vi "Windows.vi"(8 "error in (no error)":errorcluster, 10 "Font in":string, 11 "Font":refnum<vi>) -> (0 "error out":errorcluster, 2 "Font out":string)   [LabVIEW 2020]
uses:
  vi.lib/LabVIEW Icon API/lv_icon/lv_icon.lvlib
  <vilib>/registry/registry.llb/Registry SAM.ctl
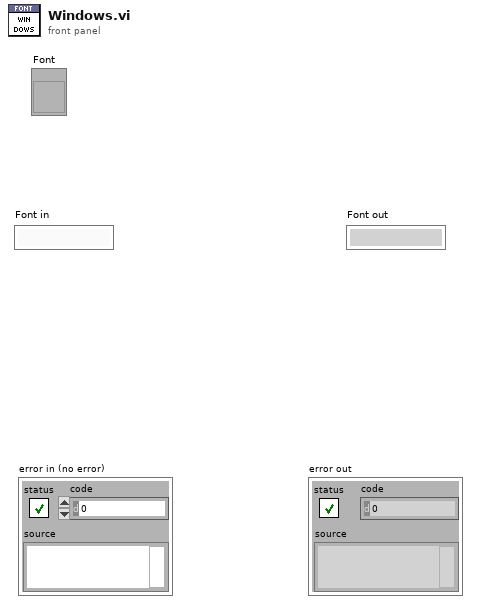
[diagram p1: front panel]
types:
  T1 = typedef "Registry SAM.ctl" = enum32{"KEY_QUERY_VALUE", "KEY_SET_VALUE", "KEY_CREATE_SUB_KEY", "KEY_ENUMERATE_SUB_KEYS", "KEY_NOTIFY", "KEY_CREATE_LINK", "KEY_READ", "KEY_WRITE", "KEY_ALL_ACCESS", "KEY_READ | KEY_WRITE"}
  T2 = typedef "Registry refnum.ctl" = refnum<k1>
  T3 = cluster{"numValues":i32, "maxValueNameLen":i32, "maxValueDataLen":i32}
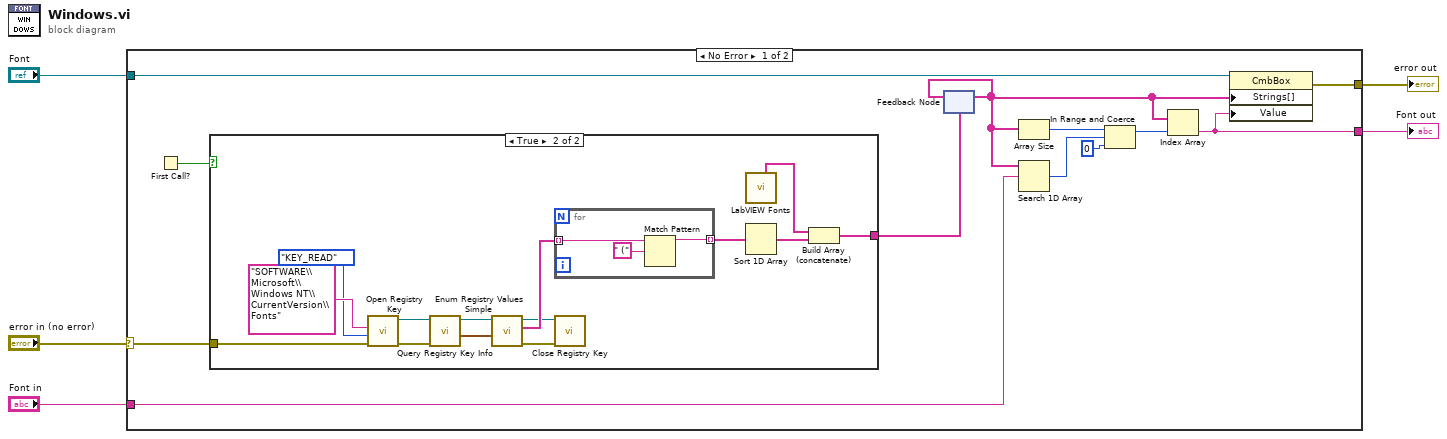
[diagram p0: block diagram]
diagram:
  n1 = case shown="No Error" "error in (no error)" {
    selector: "error in (no error)" -> [w17 w36]
    tunnel: [w16 w36] -> w4
    tunnel: "Font in" -> [w15 w35]
    tunnel: [w14 w35] -> w2
    tunnel: "Font" -> [w9 _]
    frame No Error {
      n2 = First Call?() -> (First Call?: T/F=w6:bool)
      n3 = case shown="True" w6 {
        tunnel: w17 -> [_ w23]
        tunnel: [_ w20] -> w8
        frame False {
        }
        frame True {
          n4 = call <vilib>:"Open Registry Key.vi"("error in (no error)"=w23, "security access mask (KEY_READ | KEY_WRITE)"=Registry_SAM."KEY_READ", "subkey"="SOFTWARE\\Microsoft\\Windows NT\\CurrentVersion\\Fonts") -> ("error out"=w26:errorcluster, "refnum out"=w25:T2)  [unwired: 1 in, 6 out]
          n5 = call <vilib>:"Query Registry Key Info.vi"("error in (no error)"=w26, "refnum"=w25) -> ("value info"=w27:T3, "refnum out"=w28:T2)  [unwired: 8 out]
          n6 = call <vilib>:"Enum Registry Values Simple.vi"("value info"=w27, "refnum"=w28) -> ("error out"=w29:errorcluster, "values"=w31:string[], "refnum out"=w30:T2)  [unwired: 2 in, 5 out]
          n7 = for {
            tunnel: w31 -> [w34] mode=indexing
            tunnel: [w32] -> w22 mode=indexing
            n8 = Match Pattern(string=w34, regular expression=" (") -> (before substring=w32:string)  [unwired: 4 out]
          }
          n9 = call <vilib>:"Close Registry Key.vi"("error in (no error)"=w29, "refnum"=w30) -> ()  [unwired: 6 out]
          n10 = call "LabVIEW Fonts.vi"() -> ("Additional Fonts"=w19:string[])  [unwired: 1 in, 10 out]
          n11 = Sort 1D Array(array=w22) -> (sorted array=w21:string[])
          n12 = Build Array (concatenate)(w19, w21) -> (w20:string[])
        }
      }
      n13 = feedback #1(w8) -> (w7:string[])
      n14 = feedback-in #1(w7) -> ()
      n15 = Array Size(array=w7) -> (size(s)=w10:i32)
      n16 = Search 1D Array(1D array=w7, element=w15) -> (index of element=w13:i32)  [unwired: 1 out]
      n17 = In Range and Coerce(upper limit=w10, x=w13, lower limit=0 ("x")) -> (coerced(x)=w11:i32)  [unwired: 1 out]
      n18 = Index Array(array=w7, index=w11) -> (element=w14:string)
      n19 = property class="CmbBox"(reference=w9, "Strings[]"=w7, "Value"=w14) -> (error out=w16:errorcluster)  [unwired: 1 in, 1 out]
    }
    frame Error {
    }
  }
  "error out" <- w4
  "Font out" <- w2
